vi "Disconnect.vi"(8 "error in (no error)":errorcluster, 11 "RawSocket Handler in":refnum<class "RawSocket TCP Handler.lvclass">) -> (0 "error out":errorcluster, 3 "RawSocket Handler out":refnum<class "RawSocket TCP Handler.lvclass">)   [LabVIEW 2020, in "wamplv.lvlib" / "RawSocket TCP Handler.lvclass"]
uses:
  RawSocket TCP Handler.lvclass
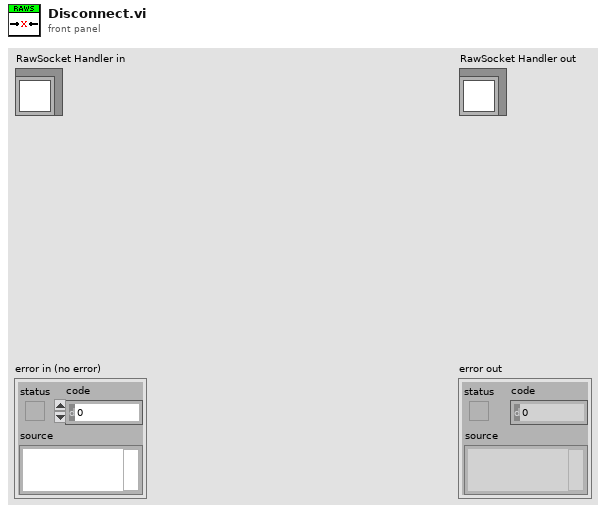
[diagram p1: front panel]
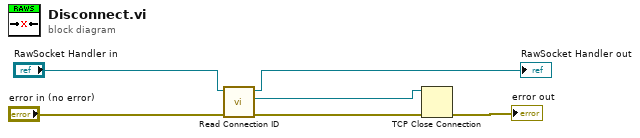
[diagram p0: block diagram]
diagram:
  n1 = call-dynamic "Read Connection ID.vi"("error in (no error)"="error in (no error)", "RawSocket Handler in"="RawSocket Handler in") -> ("error out"=w2:errorcluster, "Connection ID"=w1:refnum<k5>, "RawSocket Handler out"=→"RawSocket Handler out":refnum<class "RawSocket TCP Handler.lvclass">)  [unwired: 7 in]
  n2 = TCP Close Connection(connection ID=w1, error in (no error)=w2) -> (error out=→"error out":errorcluster)  [unwired: 1 in, 1 out]
